vi "Tiepie-Close-2018-04-26.vi"(0 "TpDeviceHandle_t":u32) -> ()   [LabVIEW 2013]
uses:
  libtiepie.dll
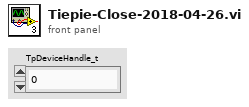
[diagram p1: front panel]
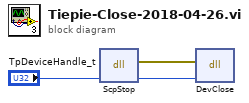
[diagram p0: block diagram]
diagram:
  n1 = dll-call lib="C:/Users/82158/Desktop/TiePieCard/libtiepie.dll" fn="ScpStop"("TpDeviceHandle_t"="TpDeviceHandle_t") -> (error out=w2:errorcluster, "TpDeviceHandle_t"=w3:u32)  [unwired: 4 in, 1 out]
  n2 = dll-call lib="C:/Users/82158/Desktop/TiePieCard/libtiepie.dll" fn="DevClose"(error in=w2, "hDevice"=w3) -> ()  [unwired: 4 in, 2 out]
